vi "Event Generate Event.vi"(4 "Video Modes":string[](array[string]), 6 "Camera Name":string, 9 "Setpoint":i64, 11 "Event Type":T1=enum."Save Data") -> ()   [LabVIEW 2023]
uses:
  Camera Set Up/Event Setup Types.ctl
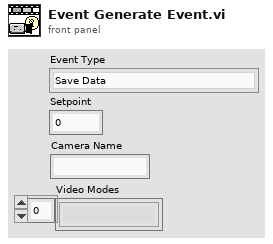
[diagram p1: front panel]
types:
  T1 = typedef "Event Setup Types.ctl" = enum16{"Default", "Camera Loop Started", "Close Settings", "GreyScale", "Open Front Panel", "Save Data", "Exit"}
  T2 = typedef "Camera Event Cluster.ctl" = cluster{"Event Type":T1, "Setpoint":i64, "Camera":string, "Video Modes":string[]}
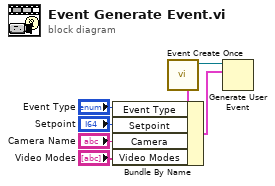
[diagram p0: block diagram]
diagram:
  n1 = call "Event Create Once.vi"() -> ("Camera Events"=w7:refnum<user-event>, "Camera Events 2"=w6:T2)  [unwired: 10 in]
  n2 = Bundle By Name(cluster=w6, "Event Type"="Event Type", "Setpoint"="Setpoint", "Camera"="Camera Name", "Video Modes"="Video Modes") -> (w5:T2)
  n3 = Generate User Event(user event=w7, event data cluster=w5) -> ()  [unwired: 2 in, 2 out]
